vi "Close.vi"(8 "error in (no error)":errorcluster, 11 "NetworkStreamWriter in":refnum<class "NetworkStreamWriter.lvclass">) -> (0 "error out":errorcluster, 3 "NetworkStreamWriter out":refnum<class "NetworkStreamWriter.lvclass">)   [LabVIEW 2011, in "NetworkStreamWriter.lvclass"]
doc: "This VI closes references internal to the NetworkStreamWriter object. This allows memory to be cleaned up effectively."
uses:
  NetworkStreamWriter.lvclass
  NetworkStreamWriter.lvclass/NetworkStreamWriter.ctl
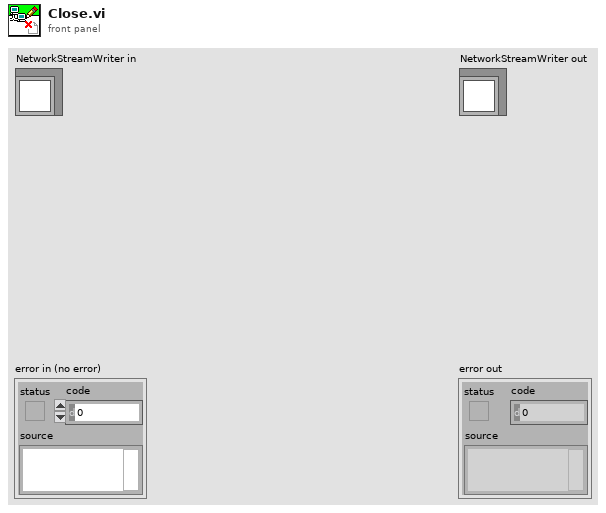
[diagram p1: front panel]
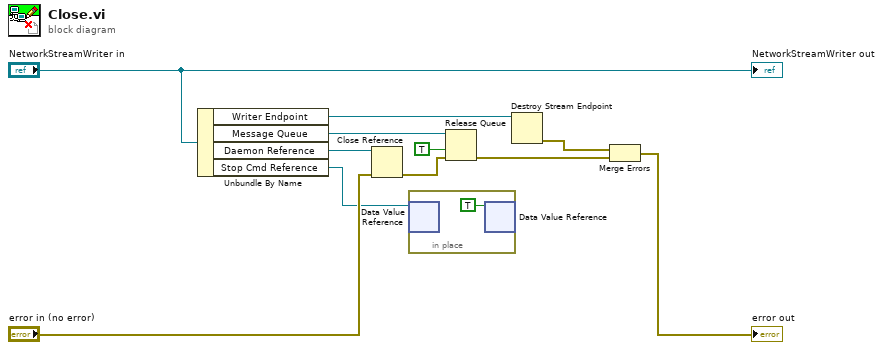
[diagram p0: block diagram]
diagram:
  n1 = Unbundle By Name("NetworkStreamWriter in") -> ("Writer Endpoint"=w6:refnum<k21>, "Message Queue"=w8:refnum<queue>, "Daemon Reference"=w9:refnum<vi>, "Stop Cmd Reference"=w4:refnum<data-value>)
  n2 = Close Reference(reference=w9, error in (no error)="error in (no error)") -> (error out=w7:errorcluster)
  n3 = in-place {
    n4 = in-place-dvr #1(w4) -> ()  [unwired: 2 out]
    n5 = in-place-dvr #1(TRUE ("data value")) -> ()  [unwired: 2 out]
  }
  n6 = Release Queue(queue=w8, force destroy? (F)=TRUE, error in (no error)=w7) -> (error out=w2:errorcluster)  [unwired: 2 out]
  n7 = Destroy Stream Endpoint(11:w6) -> (0:w3:errorcluster)  [unwired: 1 in]
  n8 = Merge Errors(w3, w2) -> (→"error out":errorcluster)
  "NetworkStreamWriter out" <- "NetworkStreamWriter in"
